vi "数据处理.vi"() -> ()   [LabVIEW 2012]
panel:
  in  "设置":refnum<vi>[](array[refnum])
  in  "布尔":bool
  in  "显示":refnum<vi>[](array[refnum])
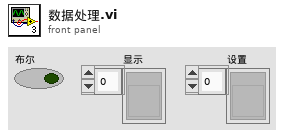
[diagram p1: front panel]
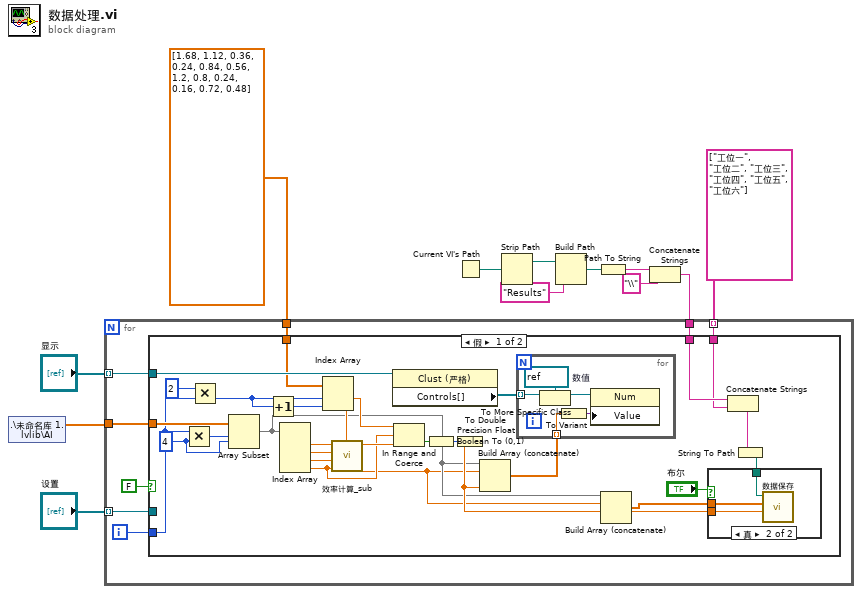
[diagram p0: block diagram]
diagram:
  n1 = shared-variable ".\\未命名库 1.lvlib\\AI"() -> (w2:dbl[])  [unwired: 1 in, 1 out]
  n2 = Current VI's Path() -> (path=w12:path)
  n3 = Strip Path(path=w12) -> (stripped path=w11:path)  [unwired: 1 out]
  n4 = Build Path(base path=w11, name or relative path="Results" ("名称或相对路径")) -> (appended path=w9:path)
  n5 = Path To String(path=w9) -> (string=w8:string)
  n6 = Concatenate Strings(w8, "\\" ("字符串")) -> (w5:string)
  n7 = for {
    tunnel: w2 -> [w20]
    tunnel: "显示" -> [w19] mode=indexing
    tunnel: dbl[] [1.68, 1.12, 0.36, 0.24, 0.84, 0.56, 1.2, 0.8, 0.24, 0.16, 0.72, 0.48] -> [w18]
    tunnel: string[] ["工位一", "工位二", "工位三", "工位四", "工位五", "工位六"] -> [w16] mode=indexing
    tunnel: w5 -> [w17]
    tunnel: "设置" -> [w13] mode=indexing
    i -> [w15]
    n8 = case shown="假" FALSE {
      tunnel: w20 -> [w48 _]
      tunnel: w19 -> [w43 _]
      tunnel: w18 -> [w42 _]
      tunnel: w17 -> [w35 _]
      tunnel: w16 -> [w34 _]
      tunnel: w15 -> [w26 _]
      tunnel: w13 -> [_ _]
      frame False {
        w47 = 4 ("y")
        n9 = Multiply(x=w26, y=w47) -> (x*y=w44:i32)
        n10 = Multiply(x=2, y=w26) -> (x*y=w40:i32)
        n11 = Array Subset(array=w48, index=w44, length=w47) -> (w24:dbl[])
        n12 = Increment(x=w40) -> (x+1=w39:i32)
        n13 = Index Array(array=w24) -> (element #1=w46:dbl, element #2=w28:dbl, element #3=w45:dbl, element #4=w29:dbl)  [unwired: 4 in]
        n14 = Index Array(array=w42, index #1=w40, index #2=w39) -> (element #1=w38:dbl, element #2=w37:dbl)
        n15 = call "效率计算_sub.vi"("输出电流"=w29, "输出电压"=w45, "输入电流"=w28, "输入电压"=w46) -> ("效率"=w23:dbl)  [unwired: 7 in]
        n16 = property class="Clust (严格)"(reference=w43) -> ("Controls[]"=w31:refnum<vi>[])  [unwired: 1 in, 2 out]
        n17 = In Range and Coerce(upper limit=w38, x=w29, lower limit=w37) -> (In Range?=w21:bool)  [unwired: 1 out]
        n18 = Boolean To (0,1)(Boolean=w21) -> (0, 1=w36:i16)
        n19 = To Double Precision Float(number=w36) -> (double precision float=w25:dbl)
        n20 = Build Array (concatenate)(w24, w23, w25) -> (w30:dbl[])  [unwired: 1 in]
        n21 = for {
          tunnel: w31 -> [w56] mode=indexing
          tunnel: w30 -> [w53] mode=indexing
          w54 = refnum<vi> refnum  # 数值
          n22 = To More Specific Class(target class=w54, reference=w56) -> (specific class reference=w55:refnum<vi>)  [unwired: 1 in, 1 out]
          n23 = To Variant(anything=w53) -> (Variant=w52:variant)
          n24 = property class="Num"(reference=w55, "Value"=w52) -> ()  [unwired: 1 in, 2 out]
        }
        n25 = Build Array (concatenate)(w24, w23) -> (w22:dbl[])  [unwired: 2 in]
        n26 = Concatenate Strings(w35, w34) -> (w33:string)
        n27 = String To Path(string=w33) -> (path=w32:path)
        n28 = case shown="真" "布尔" {
          tunnel: w25 -> [_ w51]
          tunnel: w22 -> [_ w50]
          tunnel: w32 -> [_ w49]
          frame False {
          }
          frame True {
            n29 = call "数据保存.vi"("数值"=w51, "数组"=w50, "appended path"=w49) -> ()  [unwired: 9 in]
          }
        }
      }
      frame True {
      }
    }
  }
